vi "Enqueue - Show Error Window.vi"(8 "Error In":errorcluster, 9 "Error Timestamp":timestamp, 10 "Error Message":string, 11 "Error Code":i32) -> (0 "Error Out":errorcluster)   [LabVIEW 2016, in "Error Manager.lvlib"]
doc: "Enqueues a message (a command)"
uses:
  Error Manager.lvlib
  Queues/New Error Window Loop Queue/Error Window Loop Queue.lvclass
  Queues/New Error Window Loop Queue/Command (enum).ctl
  Error Display Window/Error Details (cluster).ctl
  Error Display Window/Error Display Window.lvclass
panel:
  # "Development\ncontrols/indicators useful for development and testing, but which are not outputs of the VI"
  # "Input\nInputs to the VI"
  # "Output\nOutputs of the VI"
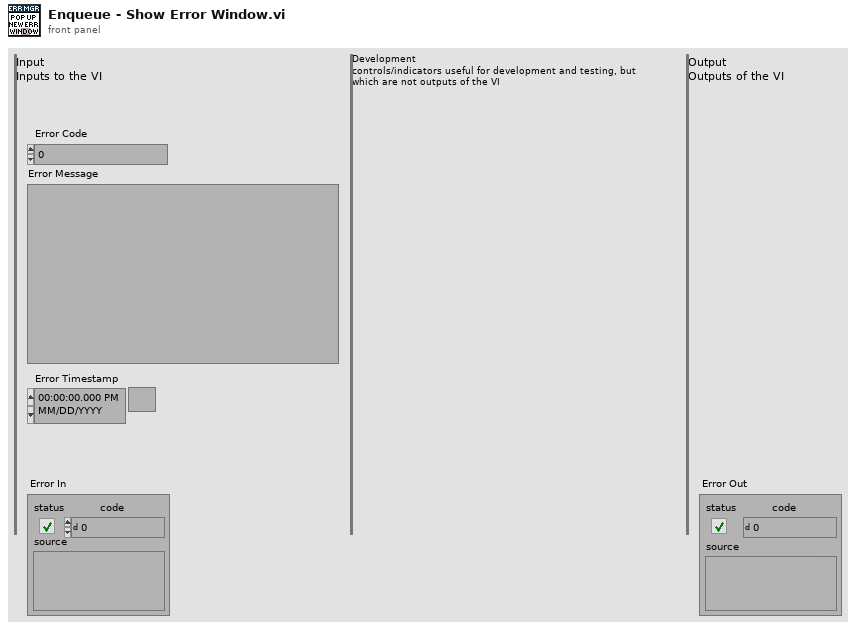
[diagram p1: front panel]
types:
  T1 = typedef "Error Manager.lvlib/Error Display Window.lvclass/Error Details (cluster).ctl" = cluster{"Error Code":i32, "Error Message":string, "Error Timestamp":timestamp}
  T2 = typedef "Error Manager.lvlib/Error Window Loop Queue.lvclass/Command (enum).ctl" = enum16{"Init Loop", "Close Loop", "Show Error Window"}
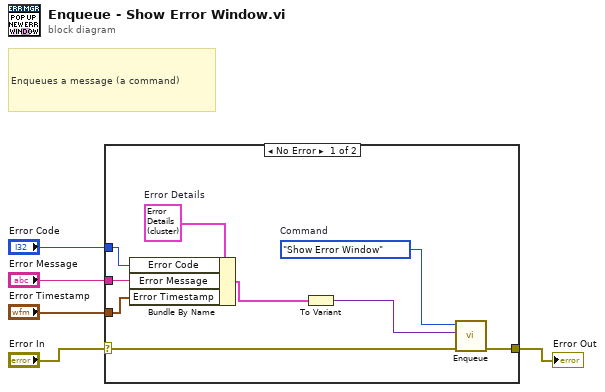
[diagram p0: block diagram]
diagram:
  # "Enqueues a message (a command)"
  n1 = case shown="No Error" "Error In" {
    selector: "Error In" -> [w14 w15]
    tunnel: [w13 w15] -> w4
    tunnel: "Error Code" -> [w8 _]
    tunnel: "Error Message" -> [w7 _]
    tunnel: "Error Timestamp" -> [w6 _]
    frame No Error {
      w10 = T1 {"Error Code"=0, "Error Message"="", "Error Timestamp"=timestamp(0 s since 1904-01-01)}  # Error Details
      w12 = Command_(enum)."Show Error Window"  # Command
      n2 = Bundle By Name(cluster=w10, "Error Code"=w8, "Error Message"=w7, "Error Timestamp"=w6) -> (w9:T1)
      n3 = To Variant(anything=w9) -> (Variant=w11:variant)
      n4 = call "Enqueue.vi"("error in (no error)"=w14, "Data"=w11, "Command"=w12) -> ("error out"=w13:errorcluster)  [unwired: 8 in]
    }
    frame Error {
    }
  }
  "Error Out" <- w4
